vi "Module.Window, Q Task.vi"(6 "Sub Panel":refnum<vi>, 7 "Q Name":string, 8 "error in":errorcluster, 9 "Show":bool, 10 "Action":T1, 11 "Q In":refnum<queue>) -> (0 "error out":errorcluster, 3 "Q Out":refnum<queue>)   [LabVIEW 2024, in "EQMF.lvlib" / "Module Utils.lvlib"]
uses:
  Module Utils.lvlib
  Queues/Q.Element.ctl
  Window.Task, Action.ctl
  _Private/Module.Window Task Data.ctl
  Queues/Queue Utils.lvlib
panel:
  # "Task=Resize, Data1 = N/A\nTask=Window, Data1 = Cmd[str], Data[Var]\n  Window(Cmd=Show Panel, Data=Show[bool])\n  Window(Cmd=Show Scroll Bars, Data=Show[bool])\n  Window(Cmd=Dock to SubPanel, Data=SubPanel[ref])\n  Window(Cmd=Undock from SubPanel, Data=N/A)\n  Window(Cmd=Return to SubPanel, Data=N/A)\nTask=Show Maint Tab, Data1 = Show[bool]\nTask=Go To Maint Tab, Data1 = N/A\nTask=Open Block Diagram, Data1 = N/A"
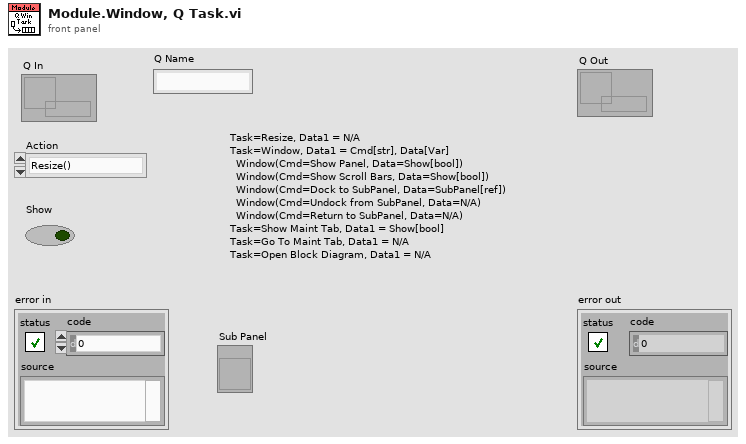
[diagram p1: front panel]
types:
  T1 = typedef "EQMF.lvlib/Module Utils.lvlib/Window.Task, Action.ctl" = enum16{"Resize()", "Show Panel(Bool)", "Show Scroll Bars(Bool)", "Dock to SubPanel(SubPanel Ref)", "Undock from SubPanel()", "Return to SubPanel()", "Go To Maint Tab()", "Show Maint Tab(Bool)", "Open Block Diagram()"}
  T2 = typedef "EQMF.lvlib/Queue Utils.lvlib/Q.Element.ctl" = cluster{"Cmd":string, "Sub":string, "Data1":variant, "Data2":variant}
  T3 = typedef "EQMF.lvlib/Module Utils.lvlib/Module.Window Task Data.ctl" = cluster{"Cmd":string, "Data":variant}
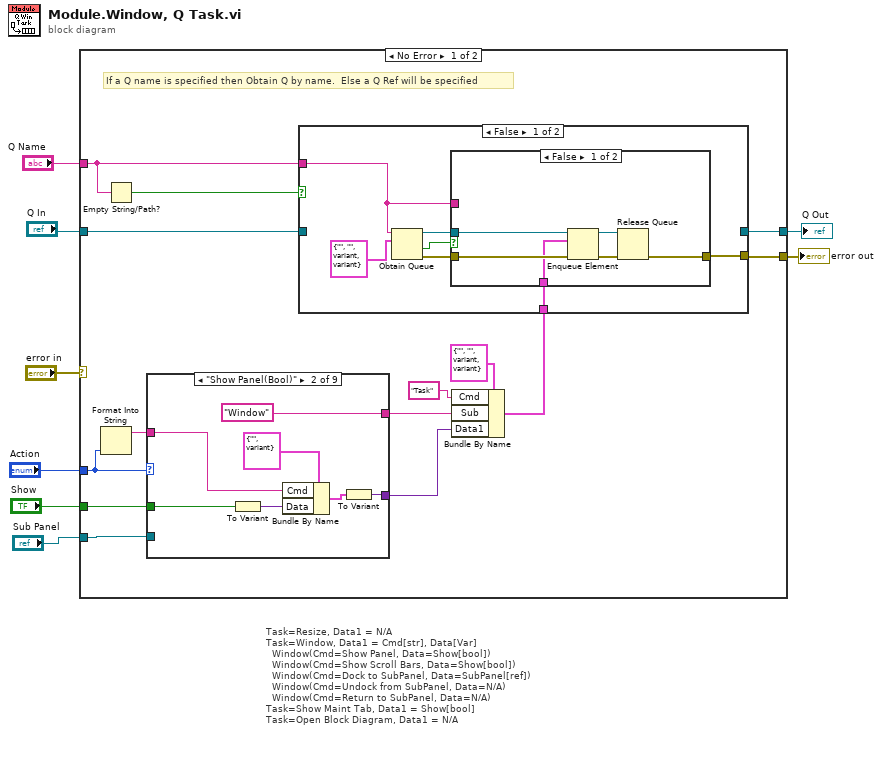
[diagram p0: block diagram]
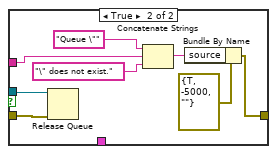
[diagram p2: hidden frame]
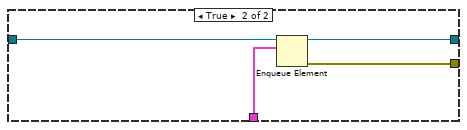
[diagram p3: hidden frame]
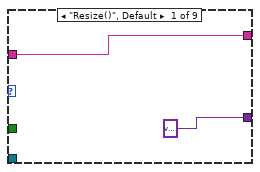
[diagram p4: hidden frame]
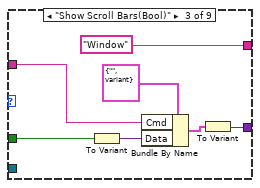
[diagram p5: hidden frame]
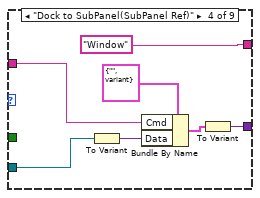
[diagram p6: hidden frame]
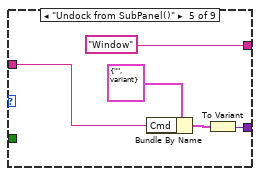
[diagram p7: hidden frame]
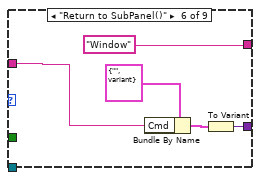
[diagram p8: hidden frame]
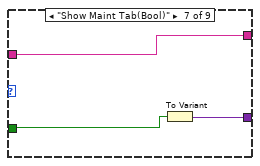
[diagram p9: hidden frame]
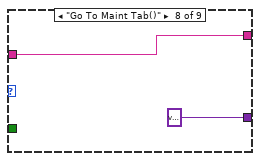
[diagram p10: hidden frame]
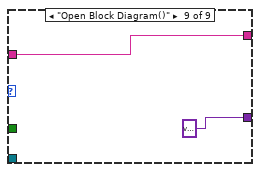
[diagram p11: hidden frame]
diagram:
  # "Task=Resize, Data1 = N/A\nTask=Window, Data1 = Cmd[str], Data[Var]\n  Window(Cmd=Show Panel, Data=Show[bool])\n  Window(Cmd=Show Scroll Bars, Data=Show[bool])\n  Window(Cmd=Dock to SubPanel, Data=SubPanel[ref])\n  Window(Cmd=Undock from SubPanel, Data=N/A)\n  Window(Cmd=Return to SubPanel, Data=N/A)\nTask=Show Maint Tab, Data1 = Show[bool]\nTask=Open Block Diagram, Data1 = N/A"
  n1 = case shown="No Error" "error in" {
    selector: "error in" -> [_ w89]
    tunnel: [w9 w89] -> w8
    tunnel: "Q In" -> [w14 w88]
    tunnel: [w10 w88] -> w5
    tunnel: "Action" -> [w18 _]
    tunnel: "Show" -> [w20 _]
    tunnel: "Sub Panel" -> [w19 _]
    tunnel: "Q Name" -> [w12 _]
    frame No Error {
      # "If a Q name is specified then Obtain Q by name.  Else a Q Ref will be specified"
      n2 = Format Into String(w18) -> (resulting string=w15:string)  [unwired: 3 in, 1 out]
      n3 = Empty String/Path?(string/path=w12) -> (empty?=w13:bool)
      n4 = case shown="\"Show Panel(Bool)\"" w18 {
        tunnel: w20 -> [_ w56 w58 _ _ _ w82 _ _]
        tunnel: w19 -> [_ _ _ w64 _ _ _ _ _]
        tunnel: [variant w51 w59 w66 w73 w77 w83 variant ("Variant") variant ("Variant")] -> w17
        tunnel: [w48 "Window" "Window" "Window" "Window" "Window" w81 w85 w86] -> w16
        tunnel: w15 -> [w48 w52 w57 w65 w71 w76 w81 w85 w86]
        frame "Resize()", Default {
        }
        frame "Show Panel(Bool)" {
          n5 = To Variant(anything=w56) -> (Variant=w53:variant)
          n6 = Bundle By Name(cluster=T3 {"Cmd"="", "Data"=variant}, "Cmd"=w52, "Data"=w53) -> (w50:T3)
          n7 = To Variant(anything=w50) -> (Variant=w51:variant)
        }
        frame "Show Scroll Bars(Bool)" {
          n8 = To Variant(anything=w58) -> (Variant=w62:variant)
          n9 = Bundle By Name(cluster=T3 {"Cmd"="", "Data"=variant}, "Cmd"=w57, "Data"=w62) -> (w61:T3)
          n10 = To Variant(anything=w61) -> (Variant=w59:variant)
        }
        frame "Dock to SubPanel(SubPanel Ref)" {
          n11 = To Variant(anything=w64) -> (Variant=w69:variant)
          n12 = Bundle By Name(cluster=T3 {"Cmd"="", "Data"=variant}, "Cmd"=w65, "Data"=w69) -> (w68:T3)
          n13 = To Variant(anything=w68) -> (Variant=w66:variant)
        }
        frame "Undock from SubPanel()" {
          n14 = Bundle By Name(cluster=T3 {"Cmd"="", "Data"=variant}, "Cmd"=w71) -> (w74:T3)
          n15 = To Variant(anything=w74) -> (Variant=w73:variant)
        }
        frame "Return to SubPanel()" {
          n16 = Bundle By Name(cluster=T3 {"Cmd"="", "Data"=variant}, "Cmd"=w76) -> (w79:T3)
          n17 = To Variant(anything=w79) -> (Variant=w77:variant)
        }
        frame "Show Maint Tab(Bool)" {
          n18 = To Variant(anything=w82) -> (Variant=w83:variant)
        }
        frame "Go To Maint Tab()" {
        }
        frame "Open Block Diagram()" {
        }
      }
      n19 = Bundle By Name(cluster=T2 {"Cmd"="", "Sub"="", "Data1"=variant, "Data2"=variant}, "Cmd"="Task", "Sub"=w16, "Data1"=w17) -> (w11:T2)
      n20 = case shown="False" w13 {
        tunnel: [w26 w47] -> w9
        tunnel: w14 -> [_ w45]
        tunnel: [_ w44] -> w10
        tunnel: w12 -> [w25 _]
        tunnel: w11 -> [w24 w46]
        frame False {
          n21 = Obtain Queue(name (unnamed)=w25, element data type=T2 {"Cmd"="", "Sub"="", "Data1"=variant, "Data2"=variant}) -> (queue out=w29:refnum<queue>, created new?=w28:bool, error out=w27:errorcluster)  [unwired: 3 in]
          n22 = case shown="False" w28 {
            tunnel: w27 -> [w31 w42]
            tunnel: w29 -> [w32 w43]
            tunnel: [w35 w37] -> w26
            tunnel: w25 -> [_ w36]
            tunnel: w24 -> [w30 _]
            frame False {
              n23 = Enqueue Element(queue=w32, element=w30, error in (no error)=w31) -> (queue out=w34:refnum<queue>, error out=w33:errorcluster)  [unwired: 1 in, 1 out]
              n24 = Release Queue(queue=w34, error in (no error)=w33) -> (error out=w35:errorcluster)  [unwired: 1 in, 2 out]
            }
            frame True {
              n25 = Release Queue(queue=w43, error in (no error)=w42) -> ()  [unwired: 1 in, 3 out]
              n26 = Concatenate Strings("Queue \"", w36, "\" does not exist.") -> (w38:string)
              n27 = Bundle By Name(cluster=errorcluster {"status"=TRUE, "code"=-5000, "source"=""} ("error constant"), "source"=w38) -> (w37:errorcluster)
            }
          }
        }
        frame True {
          n28 = Enqueue Element(queue=w45, element=w46) -> (queue out=w44:refnum<queue>, error out=w47:errorcluster)  [unwired: 2 in, 1 out]
        }
      }
    }
    frame Error {
    }
  }
  "error out" <- w8
  "Q Out" <- w5
